vi "CTRE_CANifier_GetBatteryVoltage.vi"(8 "error in":errorcluster, 11 "CANifierDevRef":T1) -> (0 "error out":errorcluster, 2 "batteryVoltage":dbl, 3 "CANifierDevRef":T1)   [LabVIEW 2017]
doc: "Get the power input voltage measurement."
uses:
  CTRE_CANifier_DeviceRef.ctl
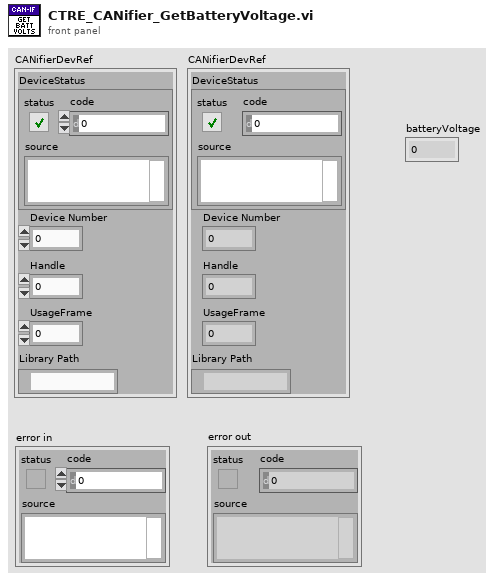
[diagram p1: front panel]
types:
  T1 = typedef "CTRE_CANifier_DeviceRef.ctl" = cluster{"DeviceStatus":errorcluster, "Device Number":u8, "Handle":u64, "UsageFrame":u32, "Library Path":path}
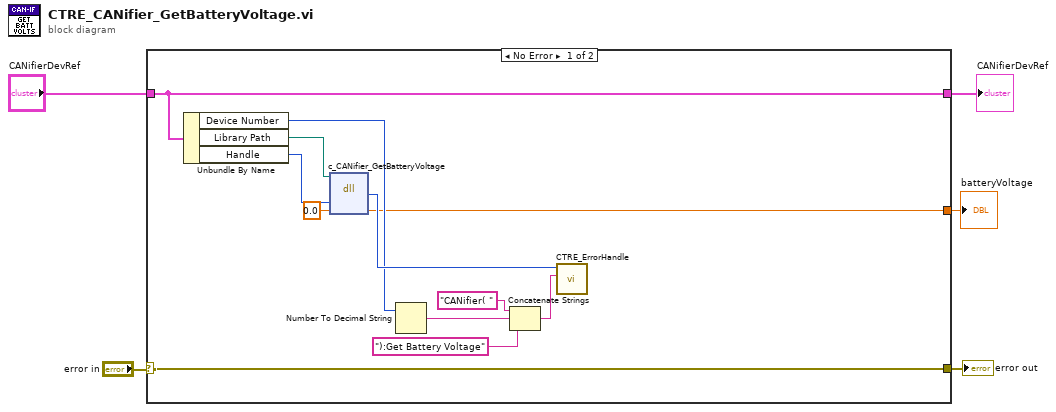
[diagram p0: block diagram]
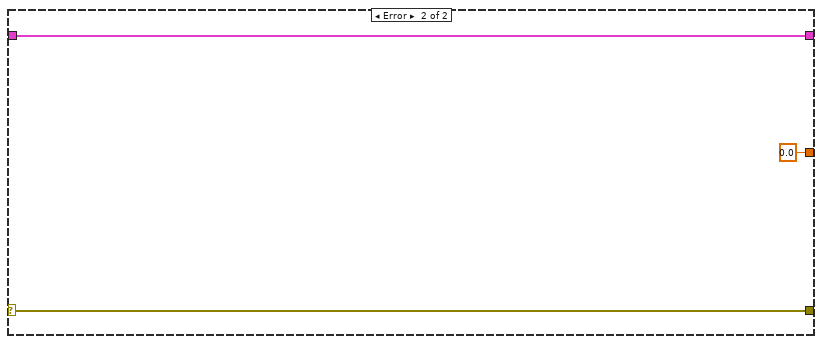
[diagram p2: hidden frame]
diagram:
  n1 = case shown="No Error" "error in" {
    selector: "error in" -> [w17 w20]
    tunnel: [w17 w20] -> w4
    tunnel: "CANifierDevRef" -> [w16 w19]
    tunnel: [w16 w19] -> w2
    tunnel: [w7 0.0 ("batteryVoltage")] -> w1
    frame No Error {
      n2 = Unbundle By Name(w16) -> ("Device Number"=w9:u8, "Library Path"=w15:path, "Handle"=w14:u64)
      n3 = dll-call lib="?" fn="c_CANifier_GetBatteryVoltage"(path in=w15, "handle"=w14, "batteryVoltage"=0.0) -> ("CTR_Code"=w13:i8, "batteryVoltage"=w7:dbl)  [unwired: 3 in, 2 out]
      n4 = Number To Decimal String(number=w9) -> (decimal integer string=w12:string)  [unwired: 1 in]
      n5 = Concatenate Strings("CANifier( " ("string"), w12, "):Get Battery Voltage" ("string")) -> (w8:string)
      n6 = call "CTRE_ErrorHandle.vi"("origin"=w8, "code"=w13) -> ()  [unwired: 9 in, 1 out]
    }
    frame Error {
    }
  }
  "error out" <- w4
  "CANifierDevRef" <- w2
  "batteryVoltage" <- w1
